vi "Finish.vi"   [LabVIEW 2016]
doc: "This VI is called just before exiting. It is expected to close I/O refnum, save collected data, etc."
uses:
  <vilib>/Rock Robotics/WPI/Utilities/WPI_GetSetVariantRefNum.vi
types:
  T1 = typedef "WPI_JoystickDevRef.ctl" = cluster{"Device":T2}
  T2 = typedef "WPI_JoystickDeviceEnum.ctl" = enum16{"USB 0", "USB 1", "USB 2", "USB 3", "USB 4", "USB 5"}
  T3 = typedef "WPI_RobotDriveDevRef.ctl" = cluster{"DevStatus":errorcluster, "Motors[]":T4[], "Square Inputs":bool, "Max Output":dbl}
  T4 = typedef "WPI_MotorControlDeviceRef.ctl" = cluster{"DeviceStatus":errorcluster, "Type":T5, "PWM":cluster{"PWM Channel":T6, "DeadBand":T7}, "CAN":cluster{"Device Number":u8, "SetOutput VI Ref":variant, "GetOutput VI Ref":variant, "Enable VI Ref":variant, "Disable VI Ref":variant, "Data":variant}, "Invert":bool}
  T5 = typedef "WPI_MotorControlType.ctl" = enum16{"PWM", "CAN"}
  T6 = typedef "FPGA_DIOPWMChannel.ctl" = enum8{"PWM 0", "PWM 1", "PWM 2", "PWM 3", "PWM 4", "PWM 5", "PWM 6", "PWM 7", "PWM 8", "PWM 9", "PWM MXP 0", "PWM MXP 1", "PWM MXP 2", "PWM MXP 3", "PWM MXP 4", "PWM MXP 5", "PWM MXP 6", "PWM MXP 7", "PWM MXP 8", "PWM MXP 9", "Invalid"}
  T7 = typedef "WPI_PWMDeadband.ctl" = cluster{"Name":string, "maxPositivePwm":i32, "minPositivePwm":i32, "centerPwm":i32, "maxNegativePwm":i32, "minNegativePwm":i32, "angularRange":u16}
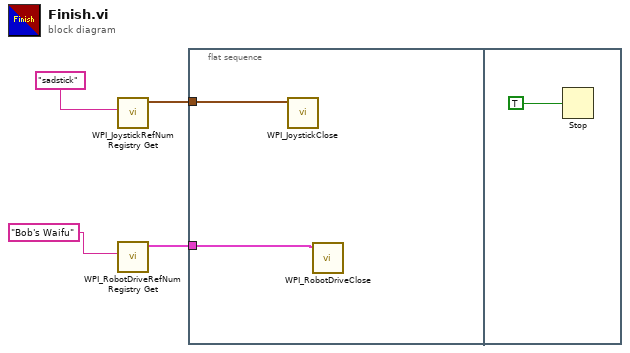
[diagram p0: block diagram]
diagram:
  n1 = call <vilib>:"WPI_JoystickRefNum Registry Get.vi"("refnum name"="sadstick") -> ("JoystickDevRef"=w3:T1)  [unwired: 1 in, 9 out]
  n2 = call <vilib>:"WPI_RobotDriveRefNum Registry Get.vi"("refnum name"="Bob's Waifu") -> ("RobotDriveDevRef"=w1:T3)  [unwired: 9 in, 1 out]
  n3 = flat-sequence {
    tunnel: w3 -> [w6]
    tunnel: w1 -> [w5]
    frame #0 {
      n4 = call <vilib>:"WPI_JoystickClose.vi"("JoystickDevRef"=w6) -> ()  [unwired: 11 out]
      n5 = call <vilib>:"WPI_RobotDriveClose.vi"("RobotDriveDevRef"=w5) -> ()  [unwired: 10 in, 1 out]
    }
    frame #1 {
      n6 = Stop(stop? (T)=TRUE ("Quit")) -> ()
    }
  }
